vi "Calculate Accel Distances.vi"(9 "Length (f)":dbl, 10 "Velocities":dbl[](array[numeric]), 11 "Limits":T2) -> (3 "Distances":T1(array[cluster]), 5 "Const V Dist":T1(array[cluster]))   [LabVIEW 2019]
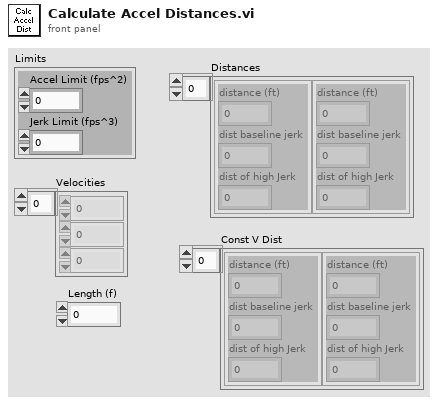
[diagram p1: front panel]
types:
  T1 = cluster{"distance (ft)":dbl, "dist baseline jerk":dbl, "dist of high Jerk":dbl}[]
  T2 = cluster{"Accel Limit (fps^2)":dbl, "Jerk Limit (fps^3)":dbl}
  T3 = cluster{"distance (ft)":dbl, "dist baseline jerk":dbl, "dist of high Jerk":dbl}
  T4 = cluster{"distance (ft)":i32, "dist baseline jerk":i32, "dist of high Jerk":i32}
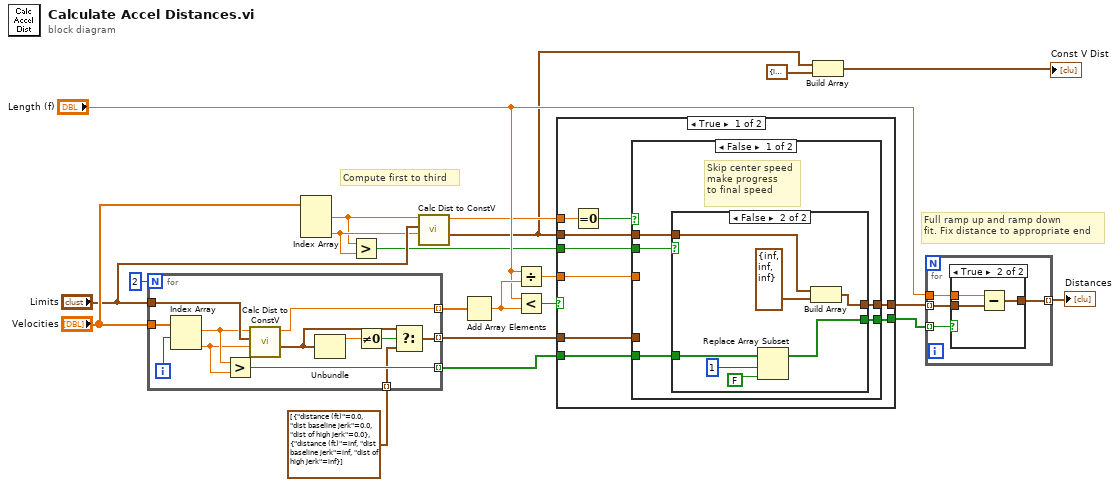
[diagram p0: block diagram]
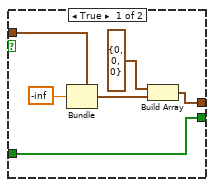
[diagram p2: hidden frame]
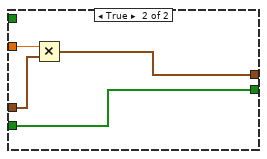
[diagram p3: hidden frame]
diagram:
  # "Compute first to third"
  # "Full ramp up and ramp down\nfit. Fix distance to appropriate end"
  n1 = for {
    N: 2 -> [_]
    tunnel: "Velocities" -> [w33]
    tunnel: "Limits" -> [w32]
    tunnel: [w29] -> w17 mode=indexing
    tunnel: [w24] -> w9 mode=indexing
    tunnel: T1 [{"distance (ft)"=0.0, "dist baseline jerk"=0.0, "dist of high Jerk"=0.0}, {"distance (ft)"=inf, "dist baseline jerk"=inf, "dist of high Jerk"=inf}] -> [w23] mode=indexing
    tunnel: [w22] -> w12 mode=indexing
    i -> [w26]
    n2 = Index Array(array=w33, index #1=w26) -> (element #1=w31:dbl, element #2=w30:dbl)  [unwired: 1 in]
    n3 = Greater?(x=w31, y=w30) -> (0:w24:bool)
    n4 = call "Calc Dist to ConstV.vi"("V2 (fps)"=w30, "Limits"=w32, "V1  (fps)"=w31) -> ("distances"=w28:T3, "distance (ft)"=w22:dbl)  [unwired: 6 in, 1 out]
    n5 = Unbundle(w28) -> ("distance (ft)"=w25:dbl)  [unwired: 2 out]
    n6 = Not Equal To 0?(x=w25) -> (x != 0?=w27:bool)
    n7 = Select(t=w28, s=w27, f=w23) -> (s? t:f=w29:T3)
  }
  n8 = Index Array(array="Velocities") -> (element #1=w2:dbl, element #3=w3:dbl)  [unwired: 3 in, 1 out]
  n9 = Greater?(x=w2, y=w3) -> (0:w1:bool)
  n10 = call "Calc Dist to ConstV.vi"("V2 (fps)"=w3, "Limits"="Limits", "V1  (fps)"=w2) -> ("distances"=w4:T3, "distance (ft)"=w7:dbl)  [unwired: 6 in, 1 out]
  n11 = Add Array Elements(numeric array=w12) -> (sum=w11:dbl)
  n12 = Divide(x="Length (f)", y=w11) -> (x/y=w18:dbl)
  n13 = Less?(x="Length (f)", y=w11) -> (x < y?=w15:bool)
  n14 = case shown="True" w15 {
    tunnel: w18 -> [w34 _]
    tunnel: w17 -> [w35 w66]
    tunnel: [w42 w66] -> w16
    tunnel: w9 -> [w40 w65]
    tunnel: [w39 w65] -> w8
    tunnel: w4 -> [w41 _]
    tunnel: w7 -> [w37 _]
    tunnel: w1 -> [w38 _]
    frame True {
      n15 = Equal To 0?(x=w37) -> (x = 0?=w36:bool)
      n16 = case shown="False" w36 {
        tunnel: [w47 w62] -> w42
        tunnel: w41 -> [w46 _]
        tunnel: w40 -> [w45 w61]
        tunnel: [w44 w61] -> w39
        tunnel: w38 -> [w43 _]
        tunnel: w35 -> [_ w63]
        tunnel: w34 -> [_ w64]
        frame False {
          # "Skip center speed\nmake progress\nto final speed"
          n17 = case shown="False" w43 {
            tunnel: [w53 w60] -> w47
            tunnel: w46 -> [w50 w59]
            tunnel: w45 -> [w48 w58]
            tunnel: [w48 w56] -> w44
            frame True {
              n18 = Bundle(cluster=w50, "dist baseline jerk"=-inf) -> (w51:T3)  [unwired: 2 in]
              n19 = Build Array(T4 {"distance (ft)"=0, "dist baseline jerk"=0, "dist of high Jerk"=0} ("distances"), w51) -> (w53:T1)
            }
            frame False {
              n20 = Replace Array Subset(array=w58, new element=FALSE, index=1) -> (w56:bool[])
              n21 = Build Array(w59, T3 {"distance (ft)"=inf, "dist baseline jerk"=inf, "dist of high Jerk"=inf} ("distances")) -> (w60:T1)
            }
          }
        }
        frame True {
          n22 = Multiply(x=w64, y=w63) -> (x*y=w62:T1)
        }
      }
    }
    frame False {
      # "Trapezoid or full triangle"
    }
  }
  n23 = Build Array(w4, T3 {"distance (ft)"=inf, "dist baseline jerk"=inf, "dist of high Jerk"=inf} ("distances")) -> (→"Const V Dist":T1)
  n24 = for {
    tunnel: w8 -> [w70] mode=indexing
    tunnel: w16 -> [w68] mode=indexing
    tunnel: "Length (f)" -> [w69]
    tunnel: [w67] -> w20 mode=indexing
    n25 = case shown="True" w70 {
      tunnel: w69 -> [_ w74]
      tunnel: w68 -> [w71 w73]
      tunnel: [w71 w72] -> w67
      frame False {
      }
      frame True {
        n26 = Subtract(x=w74, y=w73) -> (x-y=w72:T3)
      }
    }
  }
  "Distances" <- w20
